vi "openExplorer_LvPlugin.vi"() -> ()   [LabVIEW 2009]
uses:
  SHELL32.dll
panel:
  out "Path":string
  # "ツールメニューからこのVIが呼び出されると、呼び出したVIのパスを、エクスプローラで表示します。- Windows専用"
  # "ツールメニューに登録するには、LabVIEWのプログラム保存場所の projectフォルダの下にこのVIを保存するだけです。\nToolMenu Vis path : \"C:\\Program Files\\LabVIEW 2010\\project\\\""
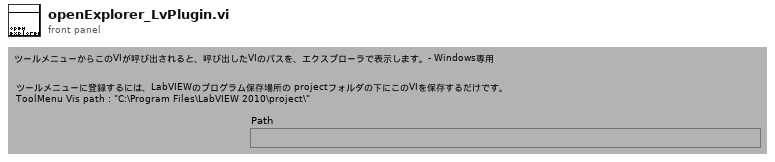
[diagram p1: front panel]
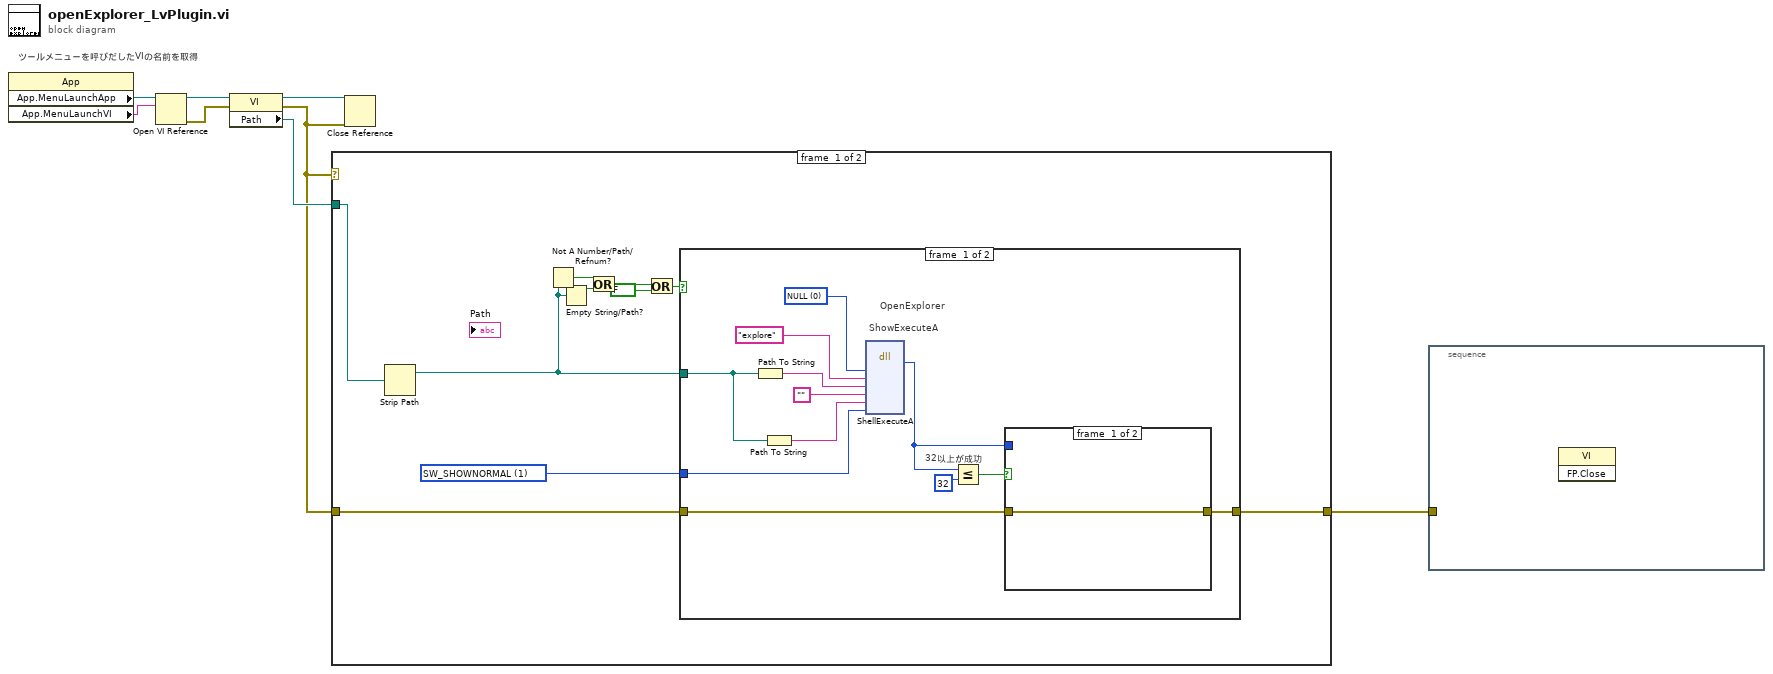
[diagram p0: block diagram]
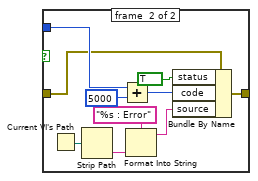
[diagram p2: hidden frame]
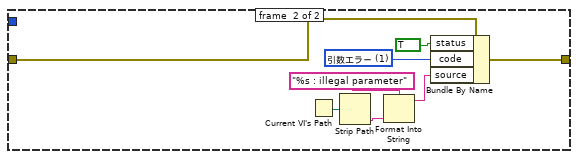
[diagram p3: hidden frame]
diagram:
  # "ツールメニューを呼びだしたVIの名前を取得"
  n1 = property class="App"() -> ("App.MenuLaunchApp"=w7:refnum<vi>, "App.MenuLaunchVI"=w8:string)  [unwired: 2 in, 2 out]
  n2 = Open VI Reference(application reference (local)=w7, vi path=w8) -> (vi reference=w6:refnum<vi>, error out=w5:errorcluster)  [unwired: 4 in]
  n3 = property class="VI"(reference=w6, error in=w5) -> (reference out=w4:refnum<vi>, error out=w2:errorcluster, "Path"=w3:path)
  n4 = case shown="エラーなし" w2 {
    tunnel: w3 -> [w11 _]
    tunnel: w2 -> [w13 w50]
    tunnel: [w12 w50] -> w1
    frame #0 {
      w10 = 1 items=["SW_HIDE", "SW_SHOWNORMAL", "SW_SHOWMINIMIZED"] ("show")
      n5 = Strip Path(path=w11) -> (stripped path=w9:path)  [unwired: 1 out]
      n6 = Not A Number/Path/Refnum?(number/path/refnum=w9) -> (NaN/Path/Refnum?=w18:bool)
      n7 = Empty String/Path?(string/path=w9) -> (empty?=w17:bool)
      n8 = Or(x=w18, y=w17) -> (x .or. y?=w16:bool)
      n9 = Or(x=w16, y=FALSE) -> (x .or. y?=w15:bool)
      n10 = case shown="FALSE" w15 {
        tunnel: [w27 w43] -> w12
        tunnel: w13 -> [w24 w44]
        tunnel: w9 -> [w21 _]
        tunnel: w10 -> [w23 _]
        frame #0 {
          w22 = 0 items=["NULL"]
          # "OpenExplorer"
          # "ShowExecuteA"
          # "32以上が成功"
          n11 = Path To String(path=w21) -> (string=w30:string)
          n12 = Path To String(path=w21) -> (string=w29:string)
          n13 = dll-call lib="SHELL32.*" fn="ShellExecuteA"("hWndParent"=w22, "lpszOp"="explore", "lpszFile"=w30, "lpszParams"="", "lpszDir"=w29, "fsShowCmd"=w23) -> ("hInstance"=w25:u32)  [unwired: 9 in, 2 out]
          n14 = Less Or Equal?(x=w25, y=u32 32) -> (x <= y?=w26:bool)
          n15 = case shown="TRUE" w26 {
            tunnel: [w31 w41] -> w27
            tunnel: w25 -> [_ w38]
            tunnel: w24 -> [w31 w36]
            frame #0 {
            }
            frame #1 {
              n16 = Current VI's Path() -> (path=w35:path)
              n17 = Strip Path(path=w35) -> (name=w32:string)  [unwired: 1 out]
              n18 = Add(x=w38, y=u32 5000) -> (x+y=w39:u32)
              n19 = Format Into String(format string="%s : Error" ("形式文字列"), w32) -> (resulting string=w33:string)  [unwired: 2 in, 1 out]
              n20 = Bundle By Name(cluster=w36, "status"=TRUE, "code"=w39, "source"=w33) -> (w41:errorcluster)
            }
          }
        }
        frame #1 {
          w49 = 1 items=["エラーなし", "引数エラー", "メモリがいっぱいです", "ゾーン外です", "ファイルの終わりです", "ファイルは既に開かれています", "一般ファイルI/Oエラー", "ファイルが見つかりません", "ファイル権限エラー", "ディスクがいっぱいです", "複製パス", "開かれているファイルが多すぎます", "システム機能が使用不可と設定されています", "リソースファイルが見つかりません", "リソースを追加できません", "リソースが見つかりません", "イメージが見つかりません", "イメージメモリエラー", "ペンが存在しません", "構成タイプが無効です", "構成トークンが見つかりません", "構成パースエラー", "構成メモリエラー", "外部コードフォーマットが無効です", "外部コードオフセットが無効です", "外部コードが存在しません", "ウィンドウがNullです", "ウィンドウの破壊エラー", "メニューがNullです", "印刷が中断されました", "印刷記録が無効です", "印刷のドライバエラー", "印刷中のウィンドウエラー", "印刷中のメモリエラー", "印刷ダイアログエラー", "一般印刷エラー", "デバイスRefnumが無効です", "デバイスが見つかりません", "デバイスのパラメータエラー", "デバイスのユニットエラー", "デバイスが開けません", "デバイスへのコールが中断されました", "一般エラー", "ユーザにより中断されました", "オブジェクトIDが低すぎます", "オブジェクトIDが高すぎます", "オブジェクトはヒープに存在しません", "不明なヒープ", "不明なオブジェクト(無効なDefProc)", "不明なオブジェクト(DefProcが表に存在しない)", "メッセージは範囲外です", "無効な（Nullな）メソッド", "不明なメッセージ", "マネージャコールはサポートされていません", "無効なアドレス", "ネットワーク操作が実行中", "ネットワーク操作がタイムアウトしました", "リソース使用中のため接続できません", "ネットワークの属性がサポートされていません", "ネットワークエラー", "アドレスが使用中です", "システムがメモリ不足です", "接続が中断されました", "接続が拒否されました", "接続していません", "既に接続しています", "接続は終了しました", "初期化エラー(インタアプリケーションマネージャ)", "無効なオカーレンス", "オカーレンスハンドルを待機中", "オカーレンスキューのオーバーフロー", "データログタイプの競合", "未使用です", "タイプを認識できません(インタアプリケーションマネージャ)", "メモリが破損しています", "一時DLLの作成に失敗しました", "CINの古いバージョンです", "ドラッグソケットが見つかりません", "ドロップオブジェクトのロードに失敗しました。", "OLEオブジェクトの登録に失敗しました", "OLEオブジェクトの開放に失敗しました", "形式の指定が一致してません", "不明な形式文字列", "形式の指定が足りません", "形式の指定が多すぎます", "スキャンに失敗しました", "新しいCINのバージョン", "バリアントへの変換エラー", "ランタイムのメニューエラー", "パスワードが変更されています", "バリアント属性は見つかりませんでした。", "不適合なバリアントデータタイプ", "イベントデータは利用できません", "イベント記憶領域は存在しません", "オカーレンスが見つかりません", "イベント待ち行列が作成されていません", "イベント情報は利用できません", "渡されたRefnumNULLです", "クラスGUIDの回収エラー", "共通クラスGUIDの回収エラー", "タイプライブラリGUIDの回収エラー", "不良アプリケーションmagicバイト", "特定のドライバは論理名に関連付けられた特定のドライバとは異なります。", "クラスドライバに対してセッションが開かれていません。", "Maxエラー", "MAX - 構成オブジェクトのエラー", "MAX - 構成のロードエラー", "MAX - グループはサポートされていません。"]
          n21 = Current VI's Path() -> (path=w47:path)
          n22 = Strip Path(path=w47) -> (name=w42:string)  [unwired: 1 out]
          n23 = Format Into String(format string="%s : illegal parameter" ("形式文字列"), w42) -> (resulting string=w45:string)  [unwired: 2 in, 1 out]
          n24 = Bundle By Name(cluster=w44, "status"=TRUE, "code"=w49, "source"=w45) -> (w43:errorcluster)
        }
      }
    }
    frame #1 {
    }
  }
  n25 = Close Reference(reference=w4, error in (no error)=w2) -> ()  [unwired: 1 out]
  n26 = stacked-sequence {
    tunnel: w1 -> [_]
    frame #0 {
      n27 = invoke class="VI" method="FP.Close"() -> ()  [unwired: 3 in, 3 out]
    }
  }
